vi "mainTest.vi"() -> ()   [LabVIEW 2018]
panel:
  out "Power On":cluster{dbl, dbl}(graph)
  in  "stop":bool
  out "RPM":dbl(knob) scale=0.0..200.0
  in  "VISA resource name":refnum<visa-resource-name>
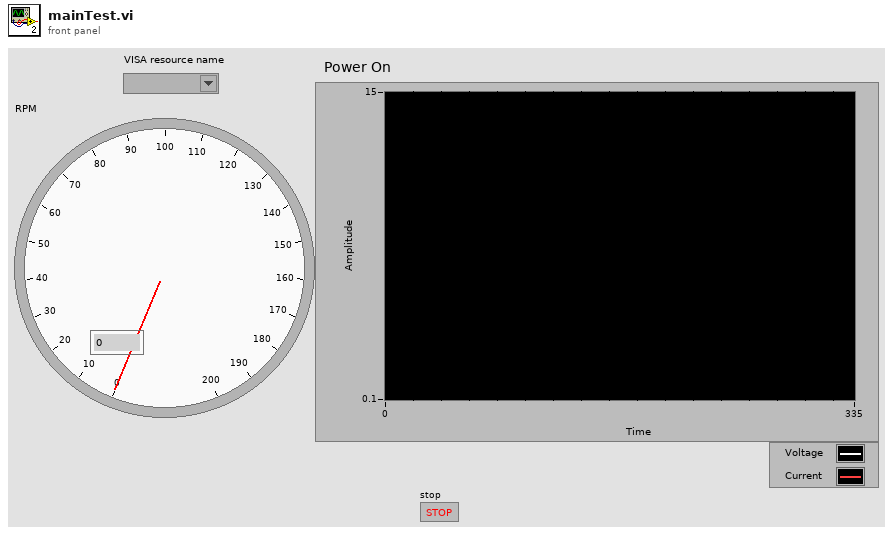
[diagram p1: front panel]
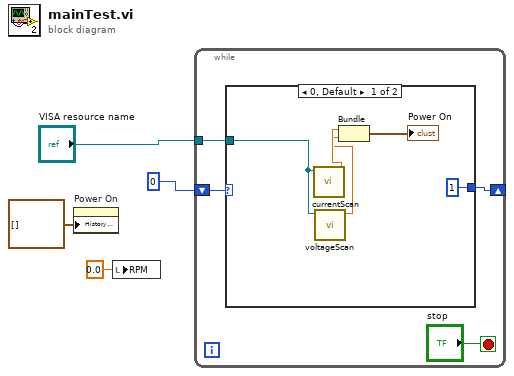
[diagram p0: block diagram]
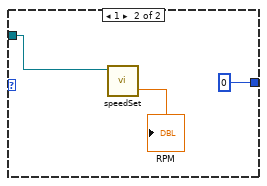
[diagram p2: hidden frame]
diagram:
  n1 = property on="Power On" class="WFChart (strict)"("History Data"=cluster{dbl, dbl}[] []) -> ()  [unwired: 2 in, 2 out]
  n2 = local write "RPM"(0.0 ("RPM")) -> ()
  n3 = while {
    tunnel: "VISA resource name" -> [w8]
    shift-right: [w6] -> _
    shift-left: 0 -> [w7]
    stop <- "stop" stop-if-true
    n4 = case shown="0, Default" w7 {
      tunnel: w8 -> [w13 w14]
      tunnel: [1 0] -> w6
      frame 0, Default {
        n5 = call "currentScan.vi"("VISA resource name"=w13) -> ("Ichart"=w10:dbl)  [unwired: 7 in, 3 out]
        n6 = call "voltageScan.vi"("VISA Refnum in"=w13) -> ("numberVoltage"=w9:dbl)  [unwired: 8 in, 2 out]
        n7 = Bundle("Ichart"=w10, "numberVoltage"=w9) -> (→"Power On":cluster{"Ichart":dbl, "\nnumberVoltage":dbl})  [unwired: 1 in]
      }
      frame 1 {
        n8 = call "speedSet.vi"("VISA resource name"=w14) -> ("RPM"=→"RPM":dbl)  [unwired: 3 in, 7 out]
      }
    }
  }
